vi "Position Data Updated.vi"(8 "error in":errorcluster, 9 "Data":variant, 10 "Point Ident":string, 11 "Task Actor in":refnum<class "Task Actor.lvclass">) -> (0 "error out":errorcluster, 3 "Task Actor out":refnum<class "Task Actor.lvclass">)   [LabVIEW 2023, in "HAL GOOP4.lvlib" / "Task Actor.lvlib" / "Task Actor.lvclass"]
uses:
  Task Actor.lvclass
  Task Actor.lvclass/Task Actor.ctl
  Task Base/Task Base.lvclass/Task Base.ctl
  Task Base/Task Base.lvclass
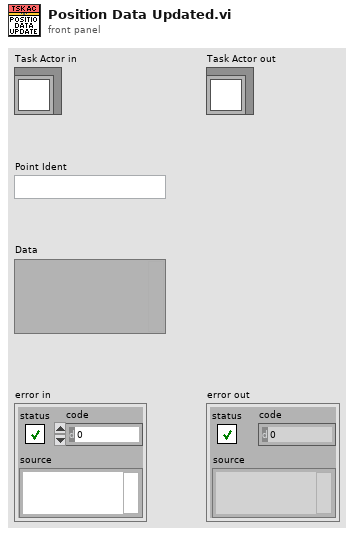
[diagram p1: front panel]
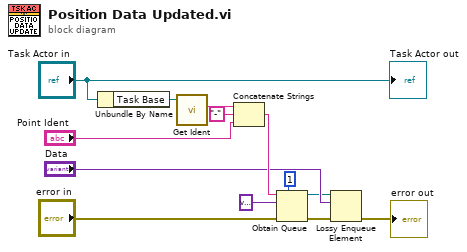
[diagram p0: block diagram]
diagram:
  n1 = Unbundle By Name("Task Actor in") -> ("Task Base"=w3:refnum<class "Task Base.lvclass">)
  n2 = call "Get Ident.vi"("Task Base in"=w3) -> ("Ident"=w2:string)  [unwired: 8 in, 2 out]
  n3 = Concatenate Strings(w2, "-" ("string"), "Point Ident") -> (w13:string)
  n4 = Obtain Queue(max queue size (-1, unlimited)=1, name (unnamed)=w13, element data type=variant, error in (no error)="error in") -> (queue out=w6:refnum<queue>, error out=w8:errorcluster)  [unwired: 1 in, 1 out]
  n5 = Lossy Enqueue Element(queue=w6, element="Data", error in (no error)=w8) -> (error out=→"error out":errorcluster)  [unwired: 3 out]
  "Task Actor out" <- "Task Actor in"
